vi "acquisitionFrameBrightness.vi"(1 "frame":u16[][](array[numeric])) -> (0 "brighness":dbl format="%0.2f")   [LabVIEW 2017]
uses:
  <vilib>/Analysis/NI_AALBase.lvlib
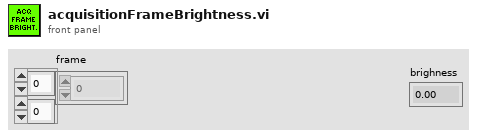
[diagram p1: front panel]
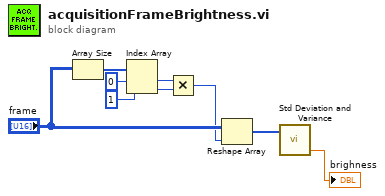
[diagram p0: block diagram]
diagram:
  n1 = Array Size(array="frame") -> (size(s)=w9:i32[])
  n2 = Index Array(array=w9, index #1=0 ("index"), index #2=1 ("index")) -> (element #1=w6:i32, element #2=w5:i32)
  n3 = Multiply(x=w6, y=w5) -> (x*y=w3:i32)
  n4 = Reshape Array("frame", w3) -> (w2:u16[])
  n5 = call <vilib>:"Std Deviation and Variance.vi"("X"=w2) -> ("variance"=→"brighness":dbl)  [unwired: 1 in, 2 out]
